vi "VC_Alignment_TA_170412.vi"() -> ()   [LabVIEW 2010]
panel:
  in  "Delay":u32
  out "Power":dbl(graph)
  out "Y position":dbl(graph)
  out "X position":dbl(graph)
  out "Position":dbl[](array[numeric])=[3.9963] format="%.6f"
  in  "Step":sgl=0.005 min=0 max=10000 format="%.3f"
  in  "End Postion":sgl=2.4 min=-400 max=400 format="%#.3f"
  in  "Start Position":sgl=3.4 min=-400 max=400 format="%#.3f"
  out "Y pos.":dbl
  out "X pos.":dbl
  out "Pow.":dbl
  in  "Launch server?":bool
  in  "Authorize?":bool=TRUE
  in  "CONEX-PSD9 Instrument Key 2":string="CONEX-PSD (A6ULD73M)"
  in  "?":bool
  in  "?":bool
  out "error out":errorcluster
  out "Identification":string="(c)2013 Physik Instrumente(PI) Karlsruhe, C-863.11,0,1.3.0.7"
  out "Conn. Axis":string[](array[string])=["1"]
  out "Running":bool caption="Mercury Setup is running"
  in  "error in":errorcluster
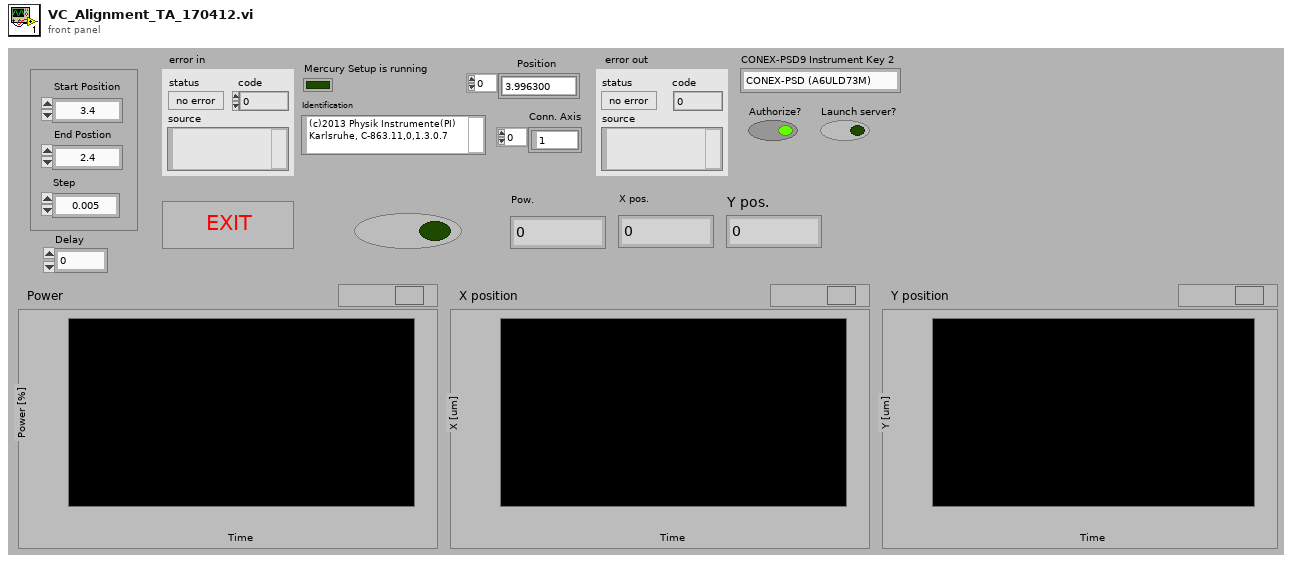
[diagram p1: front panel]
types:
  T1 = cluster{"System no.":i32, "error out":errorcluster}
  T2 = cluster{"ConexPSD Reference":refnum<k24>, "error out":errorcluster, "Component ID":i32}
  T3 = cluster{"PositionX":dbl, "PositionY":dbl, "LaserPower":dbl}
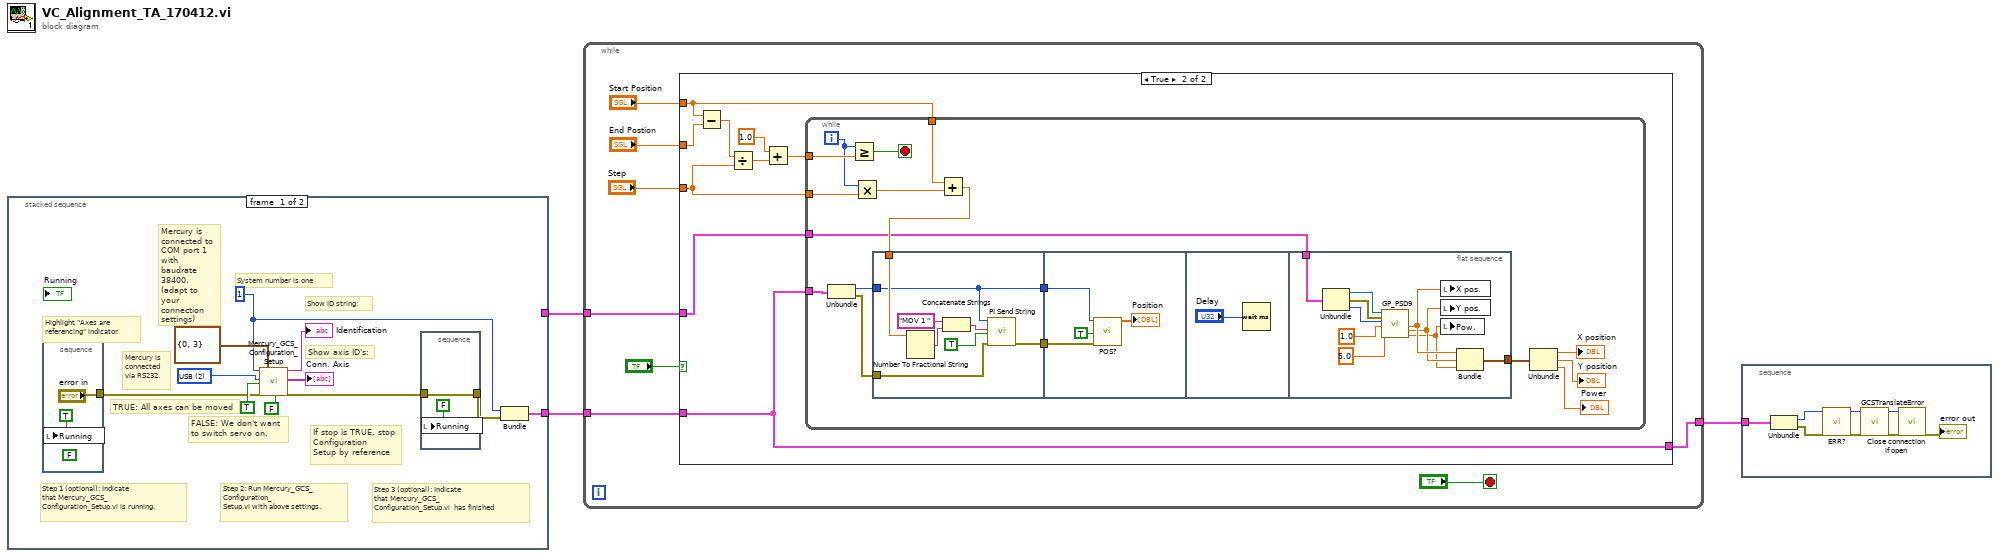
[diagram p0: block diagram]
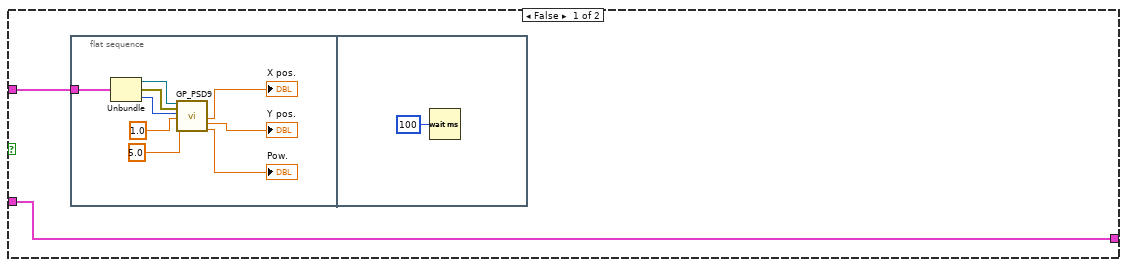
[diagram p2: hidden frame]
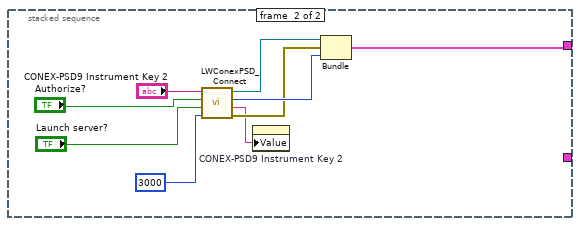
[diagram p3: hidden frame]
diagram:
  n1 = stacked-sequence {
    tunnel: [w4 _] -> w3
    tunnel: [_ w19] -> w2
    frame #0 {
      w7 = u16 2 items=["RS232", "RS232 DaisyChain", "USB", "USB_DaisyChain"] ("Interface")
      w5 = 1 ("System no.")
      # "Mercury is\nconnected\nvia RS232."
      # "If stop is TRUE, stop \nConfiguration\nSetup by reference"
      # "Mercury is\nconnected to\nCOM port 1\nwith baudrate\n38400.\n(adapt to your\nconnection\nsettings)"
      # "Step 3 (optional): Indicate\nthat Mercury_GCS_\nConfiguration_Setup.vi  has finished"
      # "Step 2: Run Mercury_GCS_\nConfiguration_\nSetup.vi with above settings."
      # "Step 1 (optional): Indicate\nthat Mercury_GCS_\nConfiguration_Setup.vi is running."
      # "Highlight \"Axes are\nreferencing\" indicator"
      # "Show axis ID's:"
      # "Show ID string:"
      # "FALSE: We don't want\nto switch servo on."
      # "TRUE: All axes can be moved"
      # "System number is one"
      n2 = stacked-sequence {
        tunnel: ["error in"] -> w10
        frame #0 {
          (unwired) FALSE ("stop")
          n3 = local write "Running"(TRUE ("Running")) -> ()
        }
      }
      n4 = call "Mercury_GCS_Configuration_Setup.vi"("System no."=w5, "Interface"=w7, "All axes?"=TRUE, "error in"=w10, "RS232 settings"=cluster{"RS232 Portnumber":i32, "Baudrate":u16} {"RS232 Portnumber"=0, "Baudrate"=3}, "Switch servo on?"=FALSE ("Use dialog to define\nconnected stages?")) -> ("Identification"=→"Identification":string, "Conn. \nAxes"=→"Conn. Axis":string[], "error out"=w11:errorcluster)  [unwired: 7 in, 4 out]
      n5 = stacked-sequence {
        tunnel: w11 -> [w18]
        tunnel: [w18] -> w6
        frame #0 {
          n6 = local write "Running"(FALSE ("Running")) -> ()
        }
      }
      n7 = Bundle("System no."=w5, "error out"=w6) -> (w4:T1)  [unwired: 1 in]
    }
    frame #1 {
      n8 = call "LWConexPSD_Connect.vi"("DiscoverTimeout (10000 msec)"=3000, "Launch server? (True)"="Launch server?", "Authorize? (True)"="Authorize?", "Instrument Key"="CONEX-PSD9 Instrument Key 2") -> ("error out"=w25:errorcluster, "Instrument Key out"=w24:string, "Component ID"=w26:i32, "ConexPSD Reference"=w22:refnum<k24>)
      n9 = property on="CONEX-PSD9 Instrument Key 2" class="Str"("Value"=w24) -> ()  [unwired: 2 in, 2 out]
      n10 = Bundle("ConexPSD Reference"=w22, "error out"=w25, "Component ID"=w26) -> (w19:T2)  [unwired: 1 in]
    }
  }
  n11 = while {
    tunnel: w3 -> [w33]
    tunnel: w2 -> [w32]
    tunnel: [w28] -> w1
    stop <- "?" stop-if-true
    n12 = case shown="True" "?" {
      tunnel: w33 -> [w36 w48]
      tunnel: w32 -> [w37 w49]
      tunnel: "Start Position" -> [_ w51]
      tunnel: "End Postion" -> [_ w56]
      tunnel: "Step" -> [_ w50]
      tunnel: [w36 w48] -> w28
      frame False {
        n13 = flat-sequence {
          tunnel: w37 -> [w38]
          frame #0 {
            n14 = Unbundle(w38) -> ("ConexPSD Reference"=w46:refnum<k24>, "error out"=w45:errorcluster, "Component ID"=w44:i32)
            n15 = call "GP_PSD9.vi"("ConexPSD Reference"=w46, "error out"=w45, "Component ID"=w44, "Adress"=1.0, "shot average"=5.0) -> ("PositionX"=→"X pos.":dbl, "PositionY"=→"Y pos.":dbl, "LaserPower"=→"Pow.":dbl)  [unwired: 8 in, 4 out]
          }
          frame #1 {
            n16 = Wait (ms)(milliseconds to wait=u32 100) -> ()  [unwired: 1 out]
          }
        }
      }
      frame True {
        n17 = Subtract(x=w51, y=w56) -> (x-y=w55:sgl)
        n18 = Divide(x=w55, y=w50) -> (x/y=w54:sgl)
        n19 = Add(x=sgl 1.0, y=w54) -> (x+y=w52:sgl)
        n20 = while {
          tunnel: w52 -> [w73]
          tunnel: w48 -> [w71]
          tunnel: w51 -> [w66]
          tunnel: w50 -> [w67]
          tunnel: w49 -> [w61]
          i -> [w68]
          stop <- w72 stop-if-true
          n21 = Unbundle(w71) -> ("System no."=w70:i32, "error out"=w69:errorcluster)
          n22 = Greater Or Equal?(x=w68, y=w73) -> (x >= y?=w72:bool)
          n23 = Multiply(x=w68, y=w67) -> (x*y=w65:sgl)
          n24 = flat-sequence {
            tunnel: w70 -> [w74]
            tunnel: w69 -> [w77]
            tunnel: w64 -> [w76]
            tunnel: [w75] -> w63
            tunnel: [w74] -> w62
            tunnel: w63 -> [w83]
            tunnel: w62 -> [w82]
            tunnel: w61 -> [w91]
            tunnel: [w87] -> w57
            frame #0 {
              n25 = Number To Fractional String(number=w76) -> (F-format string=w81:string)  [unwired: 3 in]
              n26 = Concatenate Strings("MOV 1 ", w81) -> (w78:string)
              n27 = call "PI Send String.vi"("System no."=w74, "String to send"=w78, "Attach termination char.?"=TRUE ("Attach Linefeed?"), "error in"=w77) -> ("error out"=w75:errorcluster)  [unwired: 15 in]
            }
            frame #1 {
              n28 = call "POS?.vi"("System no."=w82, "All axes?"=TRUE, "error in"=w83) -> ("Position"=→"Position":dbl[])  [unwired: 15 in, 1 out]
            }
            frame #2 {
              n29 = Wait (ms)(milliseconds to wait="Delay") -> ()  [unwired: 1 out]
            }
            frame #3 {
              n30 = Unbundle(w91) -> ("ConexPSD Reference"=w96:refnum<k24>, "error out"=w95:errorcluster, "Component ID"=w94:i32)
              n31 = call "GP_PSD9.vi"("ConexPSD Reference"=w96, "error out"=w95, "Component ID"=w94, "Adress"=1.0, "shot average"=5.0) -> ("PositionX"=w90:dbl, "PositionY"=w89:dbl, "LaserPower"=w88:dbl)  [unwired: 8 in, 4 out]
              n32 = local write "X pos."(w90) -> ()
              n33 = local write "Y pos."(w89) -> ()
              n34 = local write "Pow."(w88) -> ()
              n35 = Bundle("PositionX"=w90, "PositionY"=w89, "LaserPower"=w88) -> (w87:T3)  [unwired: 1 in]
            }
          }
          n36 = Add(x=w66, y=w65) -> (x+y=w64:sgl)
          n37 = Unbundle(w57) -> ("PositionX"=→"X position":dbl, "PositionY"=→"Y position":dbl, "LaserPower"=→"Power":dbl)
        }
      }
    }
  }
  n38 = stacked-sequence {
    tunnel: w1 -> [w99]
    frame #0 {
      n39 = Unbundle(w99) -> ("System no."=w98:i32, "error out"=w97:errorcluster)
      n40 = call "ERR?.vi"("error in"=w97) -> ("error out"=w101:errorcluster)  [unwired: 17 in, 1 out]
      n41 = call "GCSTranslateError.vi"("error in"=w101) -> ("error out"=w102:errorcluster)  [unwired: 16 in, 2 out]
      n42 = call "Close connection if open.vi"("System no."=w98, "error in"=w102) -> ("error out"=→"error out":errorcluster)  [unwired: 16 in, 1 out]
    }
  }
